vi "TDC_freezeBuffers.vi"(8 "Error In":errorcluster, 11 "Freeze":bool) -> (0 "Error Out":errorcluster)   [LabVIEW 2011]
uses:
  tdcbase.dll
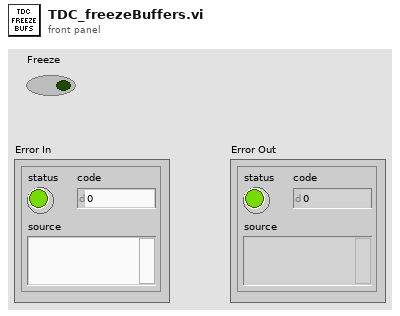
[diagram p1: front panel]
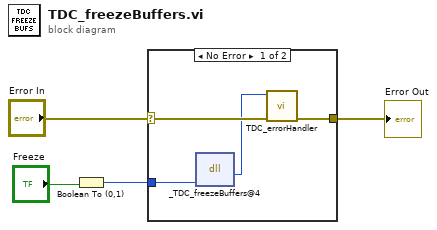
[diagram p0: block diagram]
diagram:
  n1 = Boolean To (0,1)(Boolean="Freeze") -> (0, 1=w1:i16)
  n2 = case shown="No Error" "Error In" {
    selector: "Error In" -> [w7 w9]
    tunnel: [w6 w9] -> w3
    tunnel: w1 -> [w8 _]
    frame No Error {
      n3 = dll-call lib="X:/tdcbase.dll" fn="_TDC_freezeBuffers@4"("freeze"=w8) -> ("return type"=w5:i32)  [unwired: 4 in, 2 out]
      n4 = call "TDC_errorHandler.vi"("Error In"=w7, "TDC Return Code"=w5) -> ("Error Out"=w6:errorcluster)  [unwired: 9 in]
    }
    frame Error {
    }
  }
  "Error Out" <- w3
